vi "filter.test.AddOrder.3.of.2.tickers.vi"() -> ()   [LabVIEW 2020]
uses:
  Market.Data.Common/host/fpganow.common.host.lvlib
  Market.Data.Common/fpga/orderbook.command.type.ctl
  Market.Data.Common/fpga/fpganow.common.fpga.lvlib
  Market.Data.Common/fpga/orderbook.command.ctl
panel:
  out "Metadata.Results.out":T1
  out "Data.Results.out":T4
  in  "Expected.GetState":u64[](array[numeric])=[4702127773838221344, 176, 6076284164848492576, 177, 32, 20000, 37, 20000, 48, 20000] format="%.0x"
  out "GetState":u64[](array[numeric]) format="%.0x"
  out "error out":errorcluster
  out "Debug":u64[](array[numeric]) format="%.0x"
  out "Passed":bool
  out "OrderBook.Commands.out":T2[](array[typedef]) {"symbol" format="%.0x"; "orderId" format="%.0x"; "side" format="%.0x"}
  in  "OrderBook.Commands.in":T2[](array[typedef])=[{"type"=enum."AddOrder", "side"=66, "orderId "=48, "quantity"=20000, "symbol"=4702127773838221344, "price"=9050, "executed.qty"=0, "canceled.qty"=0, "remaining.qty"=0, "seconds"=0, "nanoseconds"=0, "Add"=TRUE, "Edit"=FALSE, "Remove"=FALSE, "seq no"=10, "recv.time"=0, "parse.time"=0}, {"type"=enum."AddOrder", "side"=66, "orderId "=37, "quantity"=20000, "symbol"=4702127773838221344, "price"=9050, "executed.qty"=0, "canceled.qty"=0, "remaining.qty"=0, "seconds"=0, "nanoseconds"=0, "Add"=TRUE, "Edit"=FALSE, "Remove"=FALSE, "seq no"=11, "recv.time"=0, "parse.time"=0}, {"type"=enum."AddOrder", "side"=66, "orderId "=32, "quantity"=20000, "symbol"=6076284164848492576, "price"=9050, "executed.qty"=0, "canceled.qty"=0, "remaining.qty"=0, "seconds"=0, "nanoseconds"=0, "Add"=TRUE, "Edit"=FALSE, "Remove"=FALSE, "seq no"=12, "recv.time"=0, "parse.time"=0}]
  in  "Watch.List":string[](array[string])=["AAPL", "TSLA"]
  in  "Expected OrderBook.Commands":T2[](array[typedef])=[{"type"=enum."AddOrder", "side"=66, "orderId "=48, "quantity"=20000, "symbol"=4702127773838221344, "price"=9050, "executed.qty"=0, "canceled.qty"=0, "remaining.qty"=0, "seconds"=0, "nanoseconds"=0, "Add"=TRUE, "Edit"=FALSE, "Remove"=FALSE, "seq no"=10, "recv.time"=0, "parse.time"=0}, {"type"=enum."AddOrder", "side"=66, "orderId "=37, "quantity"=20000, "symbol"=4702127773838221344, "price"=9050, "executed.qty"=0, "canceled.qty"=0, "remaining.qty"=0, "seconds"=0, "nanoseconds"=0, "Add"=TRUE, "Edit"=FALSE, "Remove"=FALSE, "seq no"=11, "recv.time"=0, "parse.time"=0}, {"type"=enum."AddOrder", "side"=66, "orderId "=32, "quantity"=20000, "symbol"=6076284164848492576, "price"=9050, "executed.qty"=0, "canceled.qty"=0, "remaining.qty"=0, "seconds"=0, "nanoseconds"=0, "Add"=TRUE, "Edit"=FALSE, "Remove"=FALSE, "seq no"=12, "recv.time"=0, "parse.time"=0}]
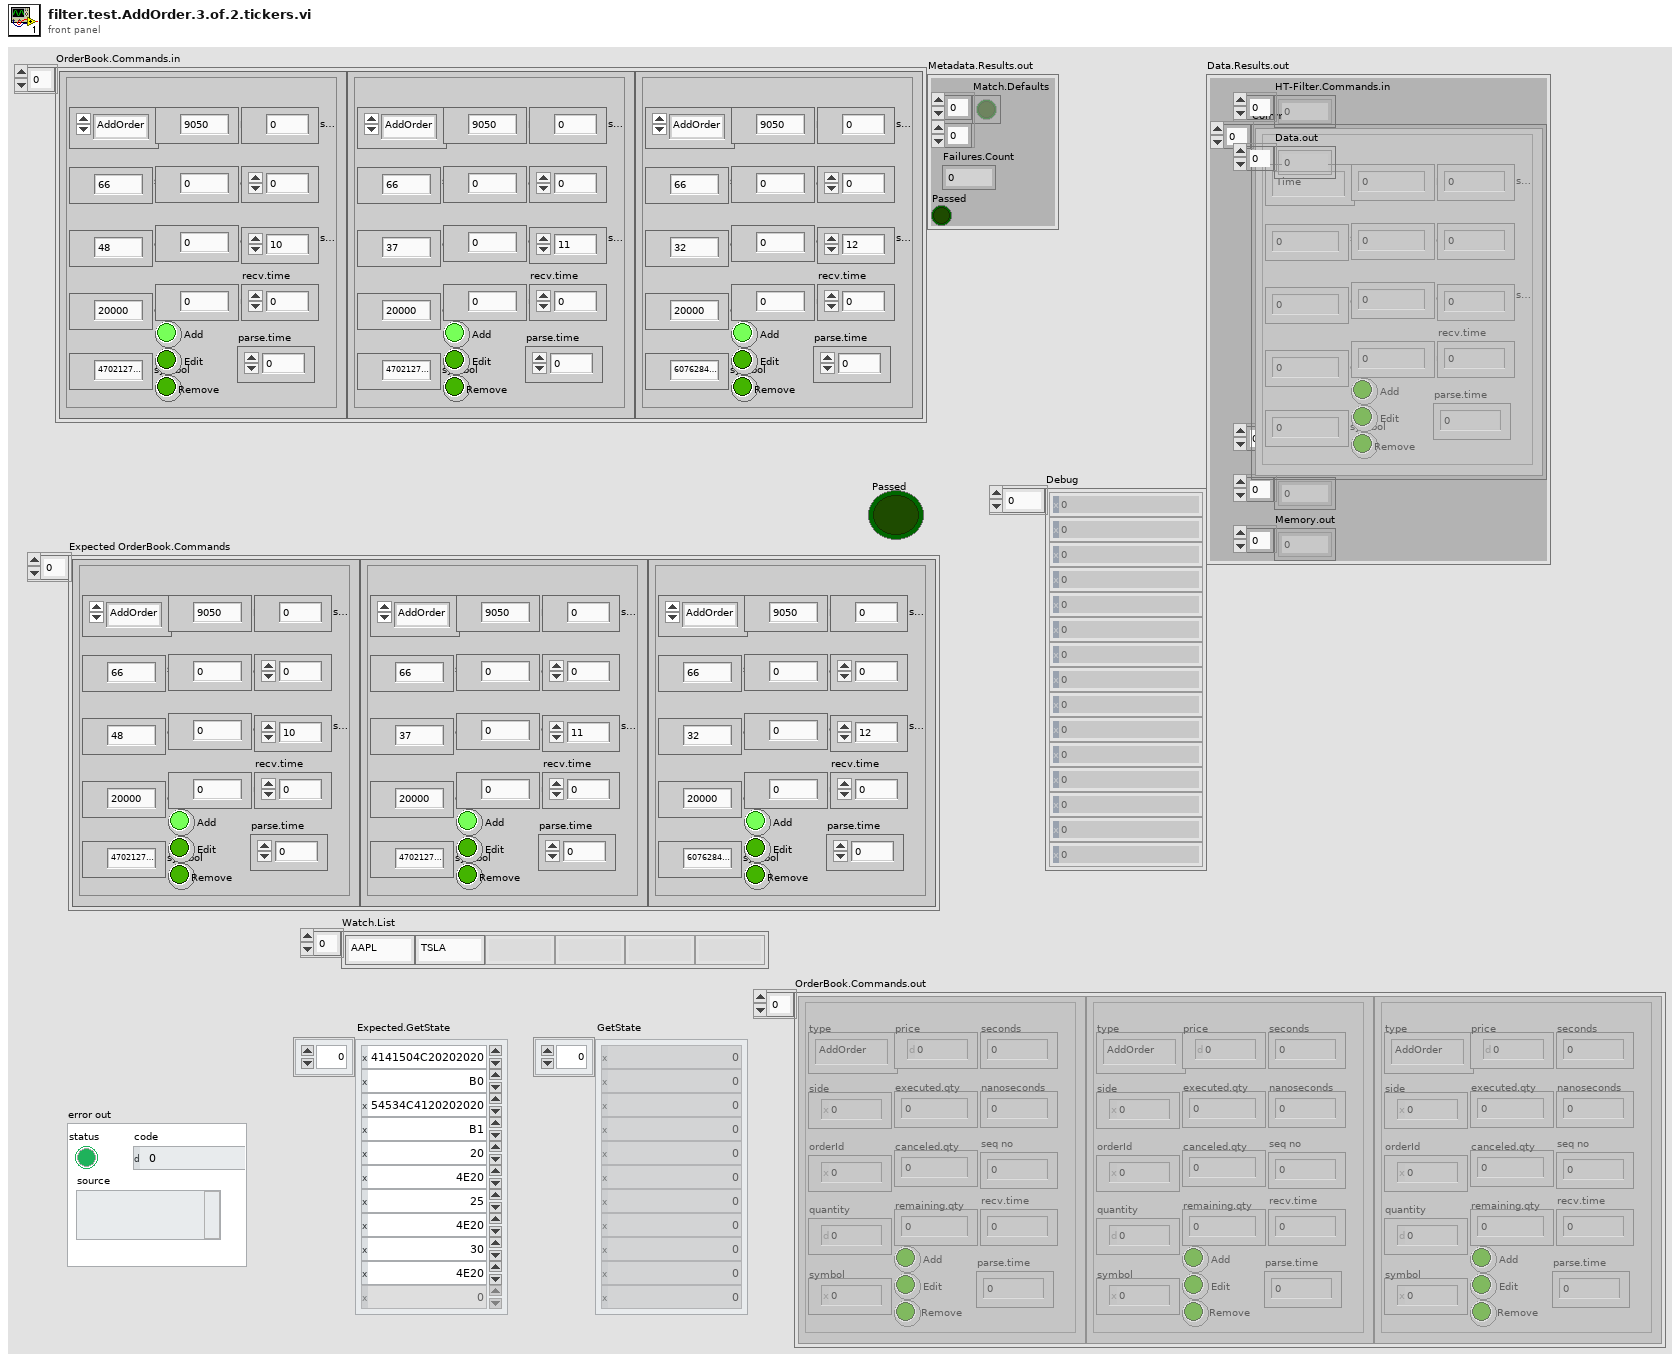
[diagram p1: front panel]
types:
  T1 = cluster{"Match.Defaults":bool[][], "Failures.Count":i32, "Passed":bool}
  T2 = typedef "fpganow.common.fpga.lvlib/orderbook.command.ctl" = cluster{"type":T3, "side":u8, "orderId ":u64, "quantity":u32, "symbol":u64, "price":u64, "executed.qty":u32, "canceled.qty":u32, "remaining.qty":u32, "seconds":u64, "nanoseconds":u64, "Add":bool, "Edit":bool, "Remove":bool, "seq no":u32, "recv.time":u64, "parse.time":u64}
  T3 = typedef "fpganow.common.fpga.lvlib/orderbook.command.type.ctl" = enum8{"Time", "AddOrder", "OrderExecuted", "OrderExecutedAtPrice", "ReduceSize", "ModifyOrder", "DeleteOrder", "Get.Everything", "Get.All.Orders", "Get.Top"}
  T4 = cluster{"HT-Filter.Commands.in":u64[], "Data.out":u64[], "Commands.out":T2[], "Debug.out":u64[], "GetState.out":u64[], "Memory.out":u64[]}
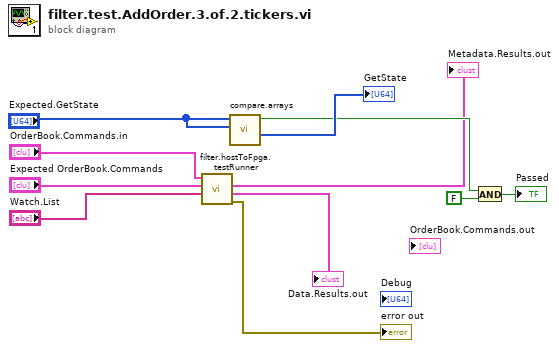
[diagram p0: block diagram]
diagram:
  n1 = call "filter.hostToFpga.testRunner.vi"("Watch.List"="Watch.List", "Expected OrderBook.Command[]"="Expected OrderBook.Commands", "OrderBook.Commands.in"="OrderBook.Commands.in") -> ("error out"=→"error out":errorcluster, "Data.Results.out"=→"Data.Results.out":T4, "Metadata.Results.out"=→"Metadata.Results.out":T1)  [unwired: 6 in]
  n2 = call "compare.arrays.vi"("Actual"="Expected.GetState", "Expected"="Expected.GetState") -> ("Actual.Out"=→"GetState":u64[], "Full.Match"=w6:bool)  [unwired: 7 in, 1 out]
  n3 = And(x=w6, y=FALSE) -> (x .and. y?=→"Passed":bool)
